vi "Incrimental Power.vi"() -> ()   [LabVIEW 2014]
panel:
  out "Motor(s) Out":dbl
  in  "Power Down":bool
  in  "Power Up":bool
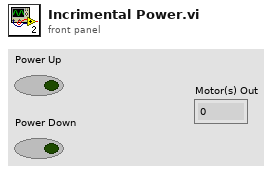
[diagram p1: front panel]
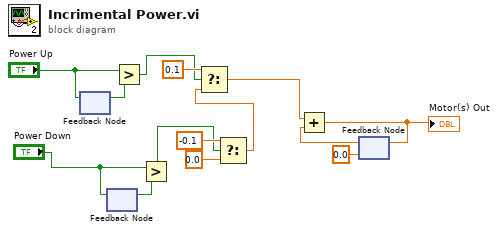
[diagram p0: block diagram]
diagram:
  n1 = feedback-in #1("Power Up") -> ()
  n2 = feedback #1() -> (w14:bool)  [unwired: 1 in]
  n3 = feedback #2() -> (w12:bool)  [unwired: 1 in]
  n4 = feedback-in #2("Power Down") -> ()
  n5 = Greater?(x="Power Up", y=w14) -> (0:w7:bool)
  n6 = Greater?(x="Power Down", y=w12) -> (0:w6:bool)
  n7 = Select(t=-0.1, s=w6, f=0.0) -> (s? t:f=w5:dbl)
  n8 = Select(t=0.1, s=w7, f=w5) -> (s? t:f=w4:dbl)
  n9 = feedback #3(0.0) -> (w2:dbl)
  n10 = Add(x=w4, y=w2) -> (x+y=w3:dbl)
  "Motor(s) Out" <- w3
  n11 = feedback-in #3(w3) -> ()
